vi "Process.vi"(8 "error in":errorcluster, 11 "MauiTemplate":refnum<class "SMO.UI.MAUI.BasicTemplate.lvclass">) -> (0 "error out":errorcluster, 3 "MauiTemplate out":refnum<class "SMO.UI.MAUI.BasicTemplate.lvclass">)   [LabVIEW 2019, in "SMO.UI.MAUI.BasicTemplate.lvclass"]
doc: "---------------------------------------------------------------\nJKI State Machine Objects™\nhttp://jki.net/state-machine-objects/\nCopyright (C) 2005-2015, JKI <info@jki.net>\nALL RIGHTS RESERVED"
uses:
  SMO.UI.MAUI.BasicTemplate.lvclass
  C:/Program Files (x86)/National Instruments/LabVIEW 2019/vi.lib/JKI/JKI SMO/SMO/SMO.lvclass
  C:/Users/patrick/Documents/GitHub/MAUI-Engine/lvsrc/Maui 1.0/SMO.UI.MAUI/SMO.UI.MAUI.lvclass
  C:/Program Files (x86)/National Instruments/LabVIEW 2019/vi.lib/JKI/JKI SMO/SMO.UI/SMO.UI.lvclass
  <vilib>/JKI/JKI SMO/SMO/Typedefs/Parent Call--Enum.ctl
  <vilib>/JKI/JKI SMO/SMO/SMO.lvclass/SMO.ctl
  Maui 1.0/SMO.UI.MAUI/Typedefs/PanelData.ctl
  <vilib>/JKI/JKI SMO/SMO/Private/ReftoDVR--SMO.vi
  Maui 1.0/SMO.UI.MAUI/SMO.UI.MAUI.lvclass
  <vilib>/JKI/JKI SMO/SMO/SMO.lvclass
  <vilib>/JKI/JKI SMO/SMO.UI/SMO.UI.lvclass
panel:
  out "Title":string
  in  "Right Ring":u16(ring)
  in  "Left Ring":u16(ring)
  # "For instructions on how to use the JKI State Machine Objects, examples and video tutorials, visit:\nhttp://jki.net/state-machine-objects/\n\nJKI State Machine Objects™\nhttp://jki.net/state-machine-objects/\nCopyright (C) 2005-2015, JKI <info@jki.net>\nALL RIGHTS RESERVED"
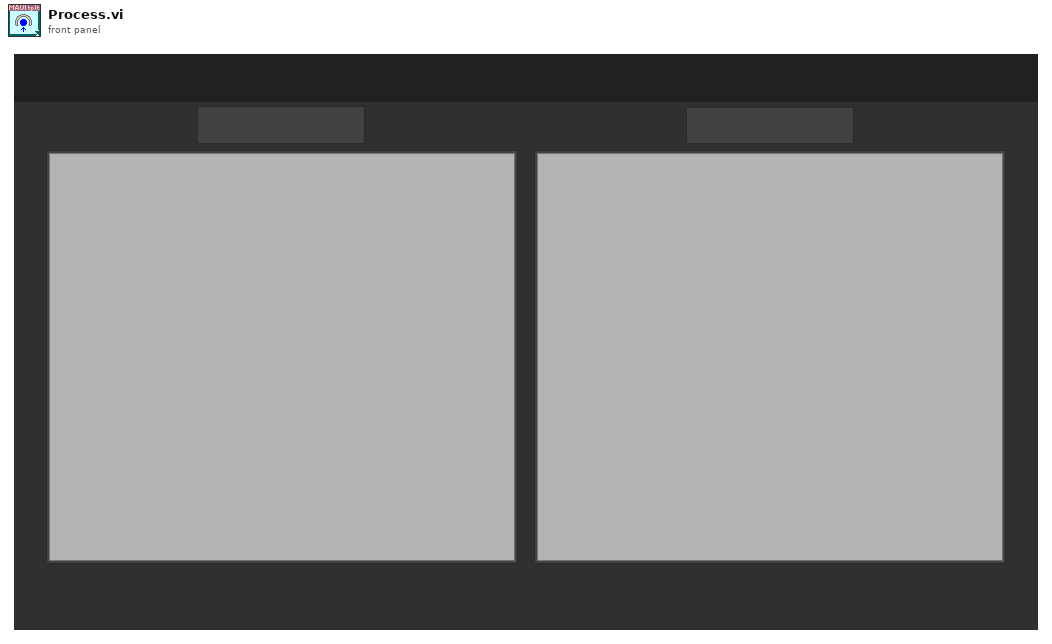
[diagram p1: front panel]
types:
  T1 = typedef "SMO.lvclass/Parent Call--Enum.ctl" = enum16{"Allows parent to run", "Does not request parent to run"}
  T2 = enum32{"invalid app kind", "Development System", "Run Time System", "Student Edition", "Embedded LabVIEW", "Evaluation", "Custom"}
  T3 = enum32{"Invalid", "Standard", "Closed", "Hidden", "Minimized", "Maximized"}
  T4 = enum32{"Bad", "Idle", "Run top level", "Running"}
  T5 = cluster{"Core":cluster{"Current VI Reference":refnum<vi>, "Close Panel on Exit?":bool, "error":errorcluster}, "MAUI":cluster{"Active Index":i32, "Panel Index":i32}, "Self Reference":refnum<class "SMO.UI.MAUI.BasicTemplate.lvclass">}
  T6 = cluster{"Current VI Reference":refnum<vi>, "Close Panel on Exit?":bool, "error":errorcluster}
  T7 = typedef "SMO.lvclass/Protected Events.ctl" = cluster{"StopProcesses":refnum<user-event>, "AbortProcesses":refnum<user-event>, "Config Changed":refnum<user-event>, "Dependency":refnum<user-event>}
  T8 = typedef "SMO.UI.MAUI.lvclass/PublicEvents--Cluster.ctl" = cluster{"ReadyForInfo ":refnum<user-event>}
  T9 = typedef "SMO.UI.MAUI.lvclass/PanelData.ctl" = cluster{"SubPanel":refnum<vi>, "Ring":refnum<vi>, "Active":i32}
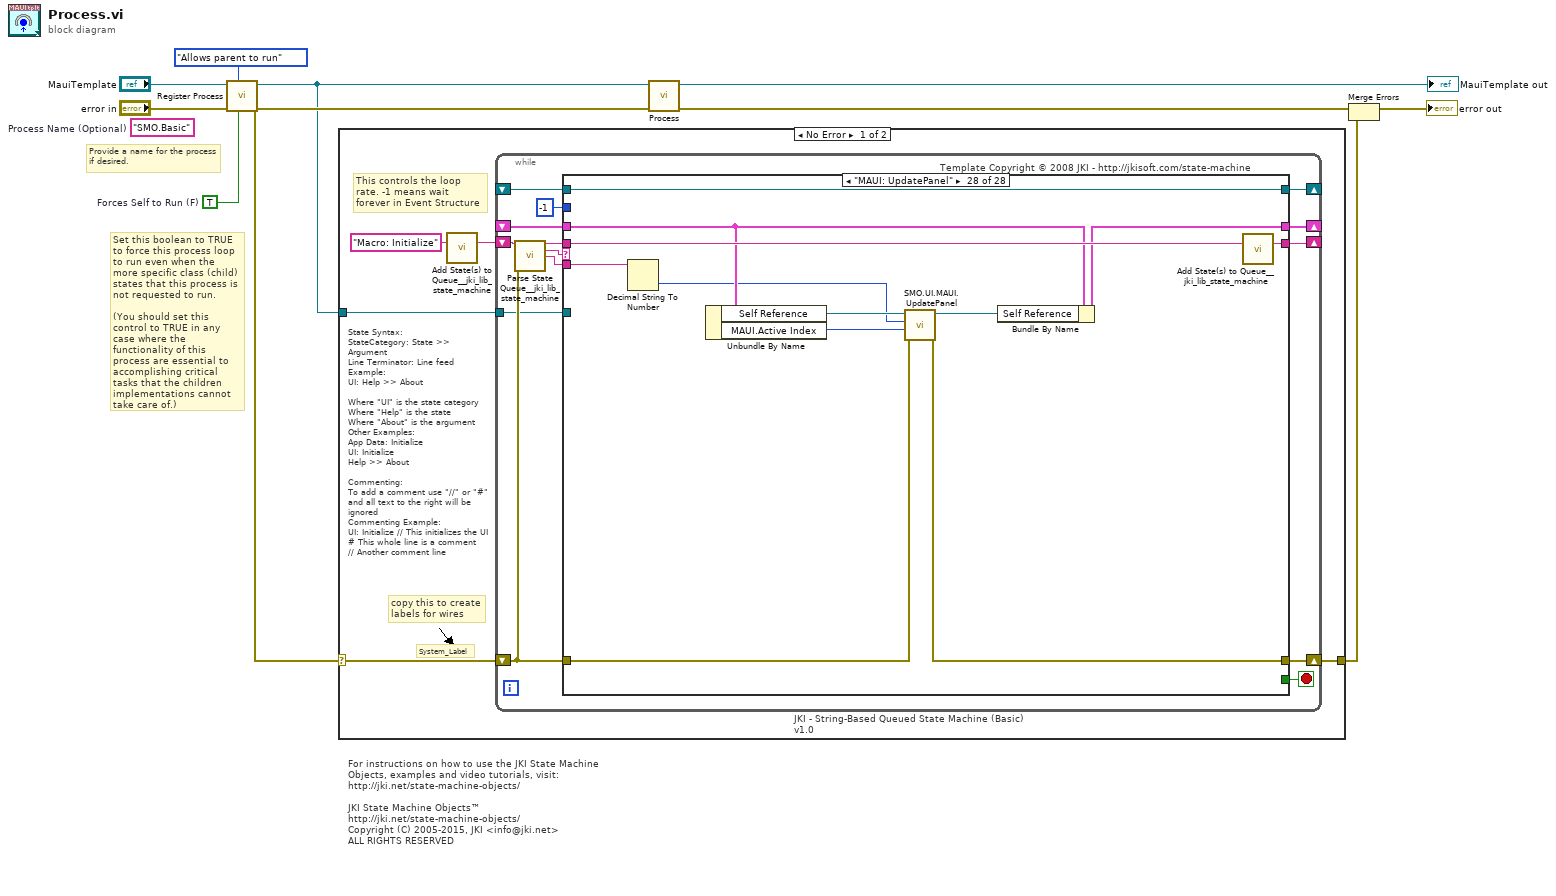
[diagram p0: block diagram]
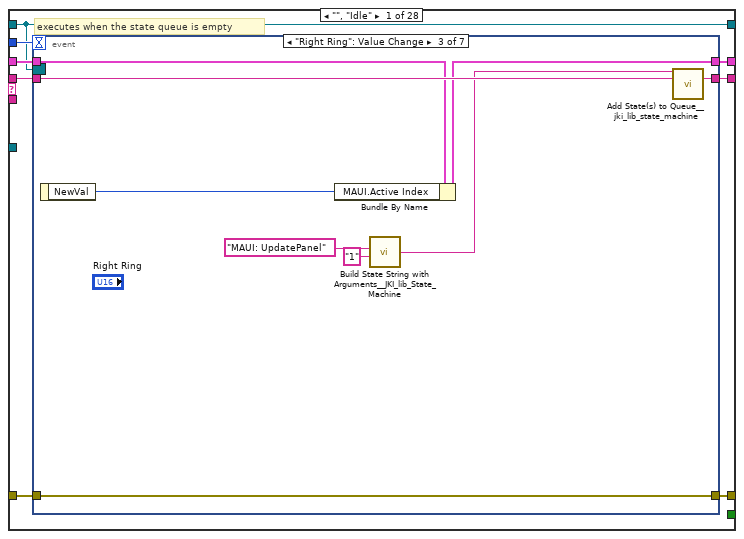
[diagram p2: hidden frame]
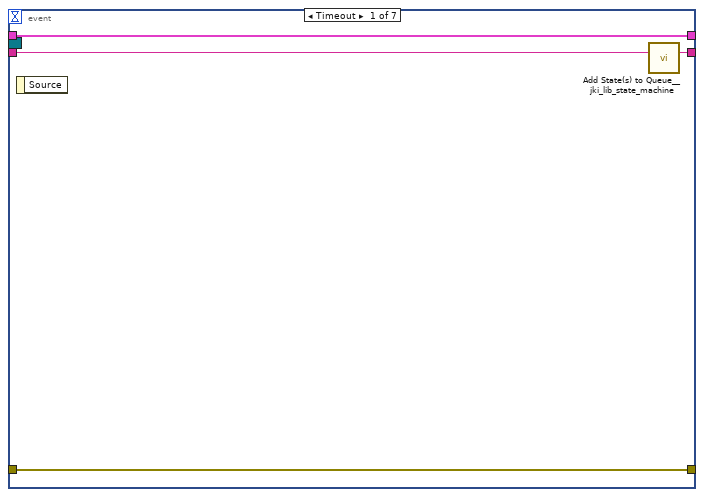
[diagram p3: hidden frame]
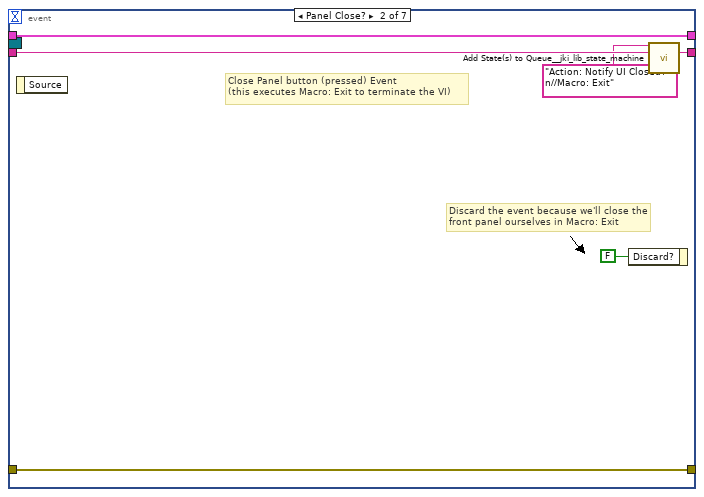
[diagram p4: hidden frame]
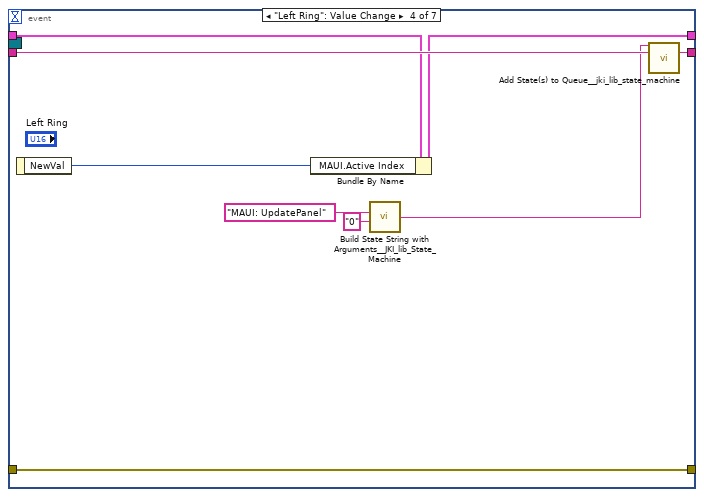
[diagram p5: hidden frame]
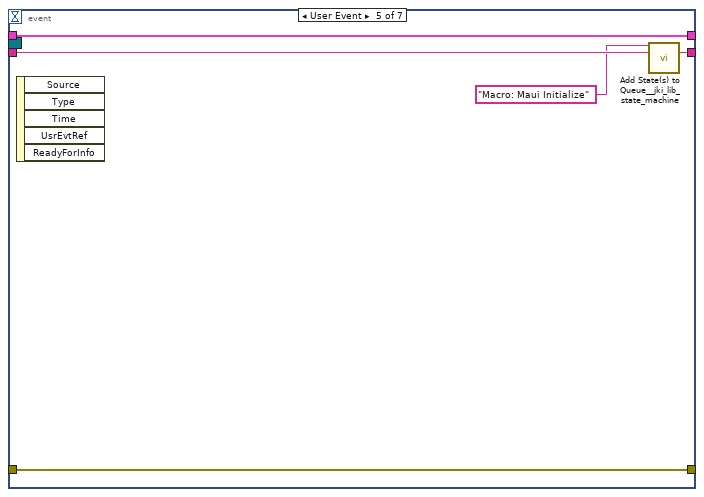
[diagram p6: hidden frame]
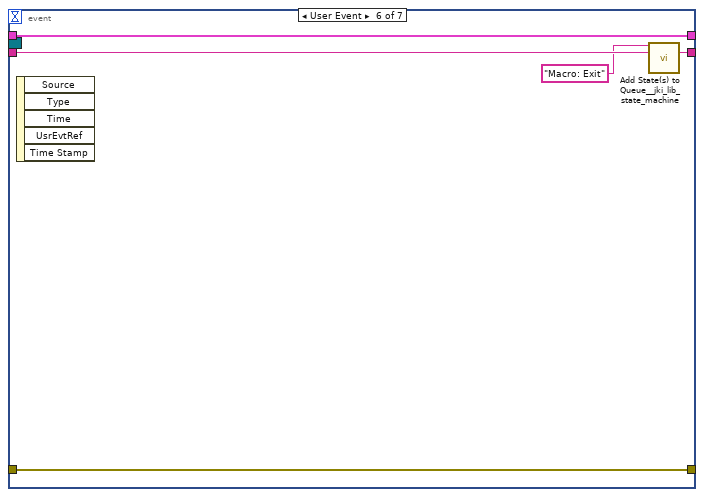
[diagram p7: hidden frame]
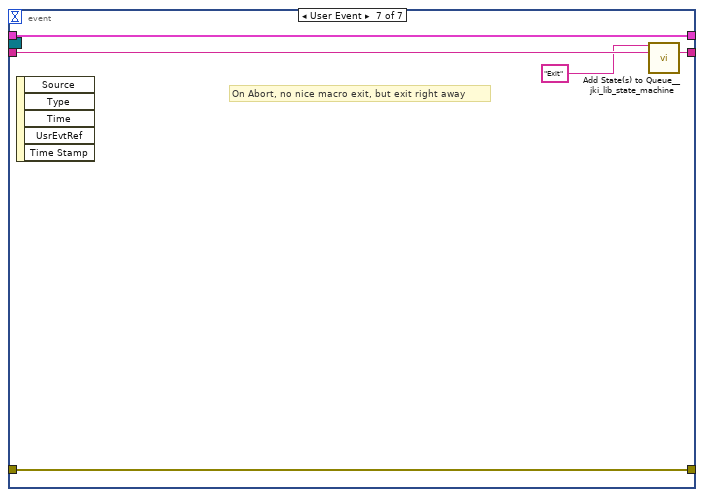
[diagram p8: hidden frame]
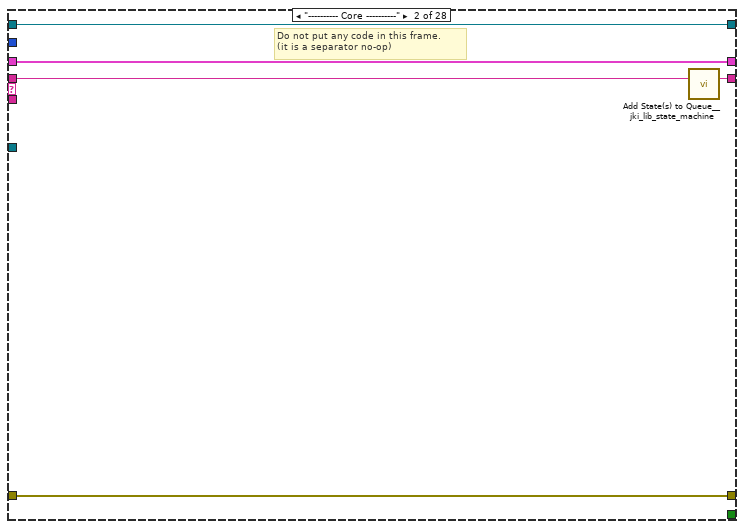
[diagram p9: hidden frame]
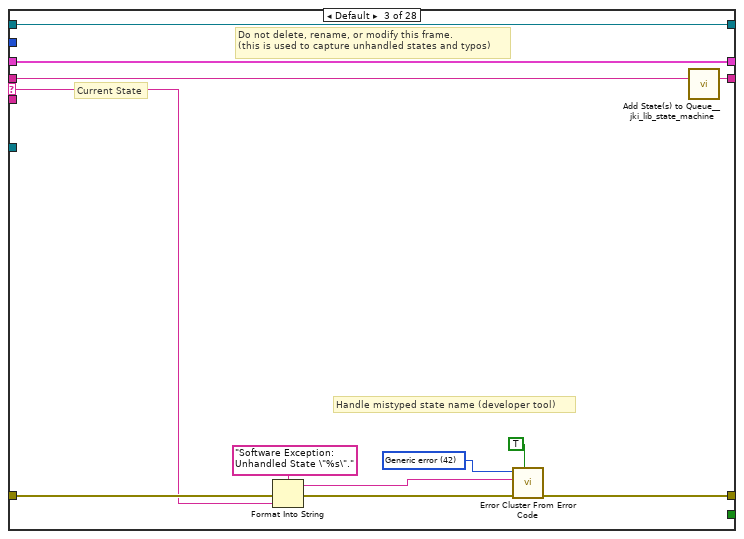
[diagram p10: hidden frame]
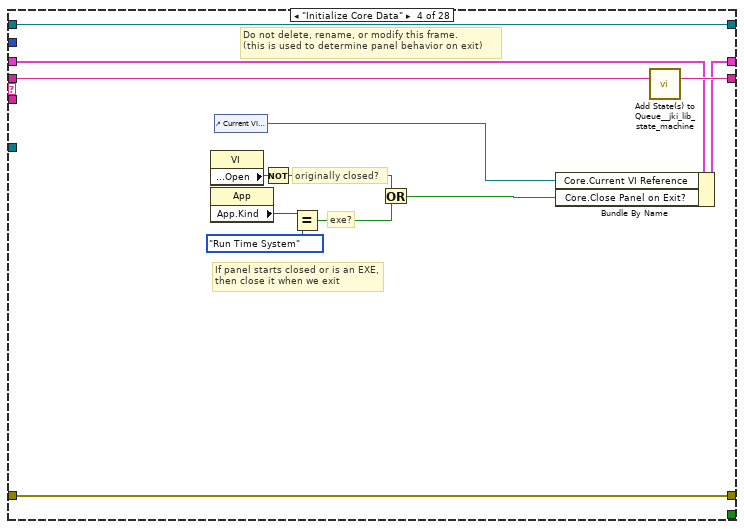
[diagram p11: hidden frame]
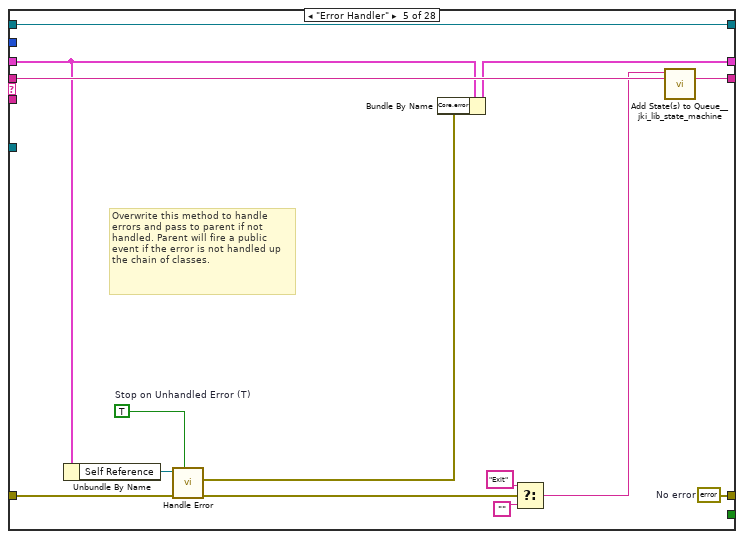
[diagram p12: hidden frame]
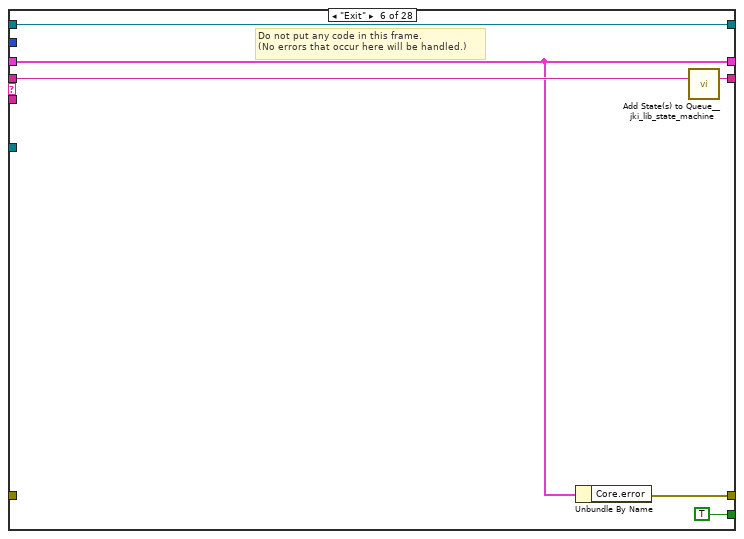
[diagram p13: hidden frame]
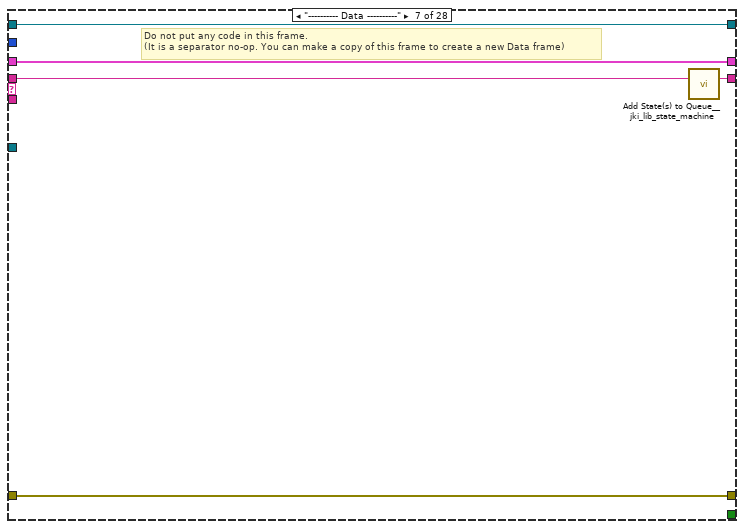
[diagram p14: hidden frame]
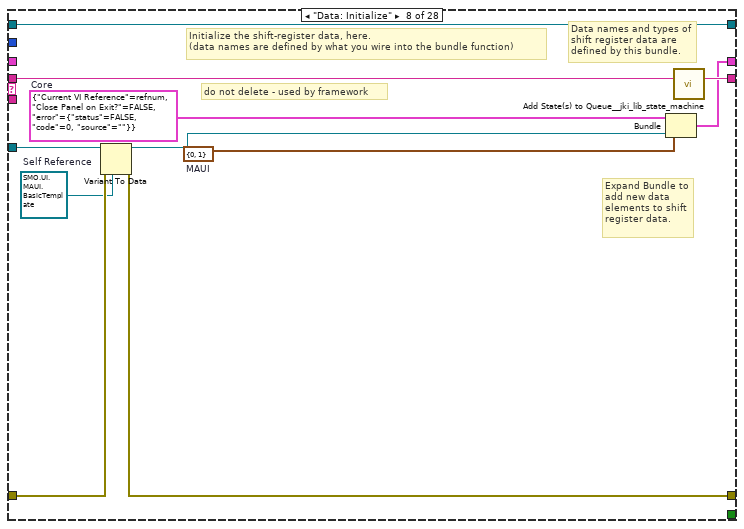
[diagram p15: hidden frame]
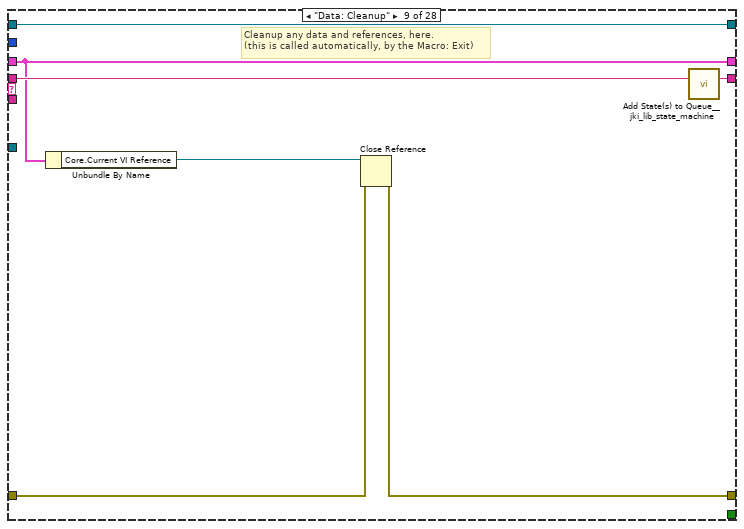
[diagram p16: hidden frame]
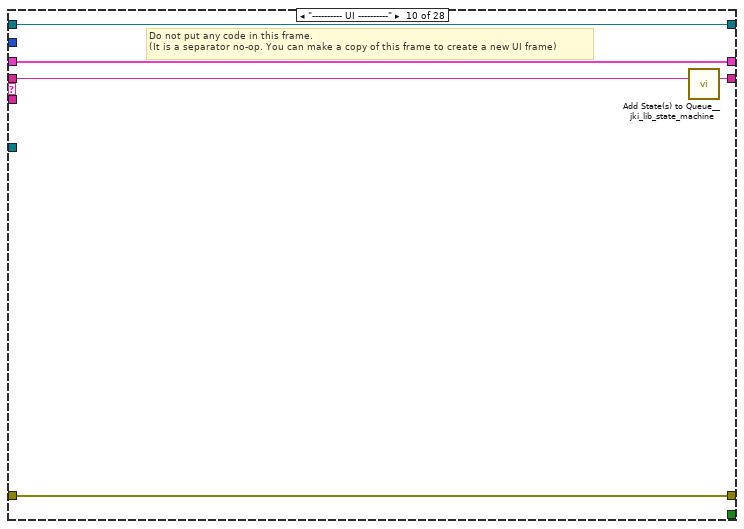
[diagram p17: hidden frame]
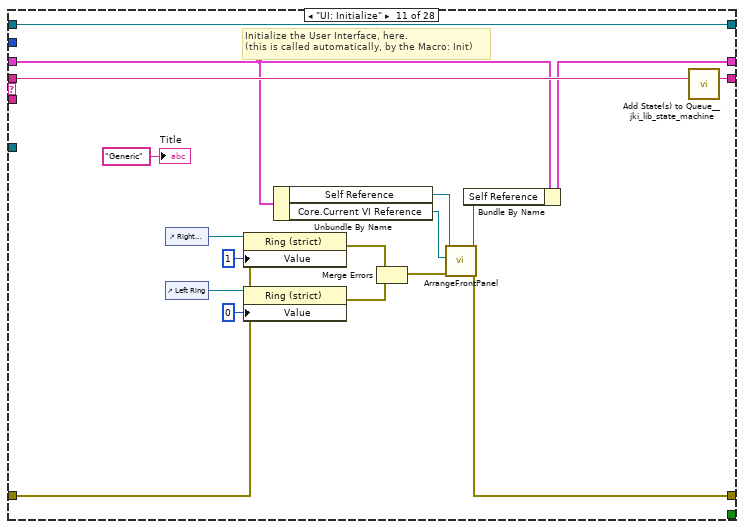
[diagram p18: hidden frame]
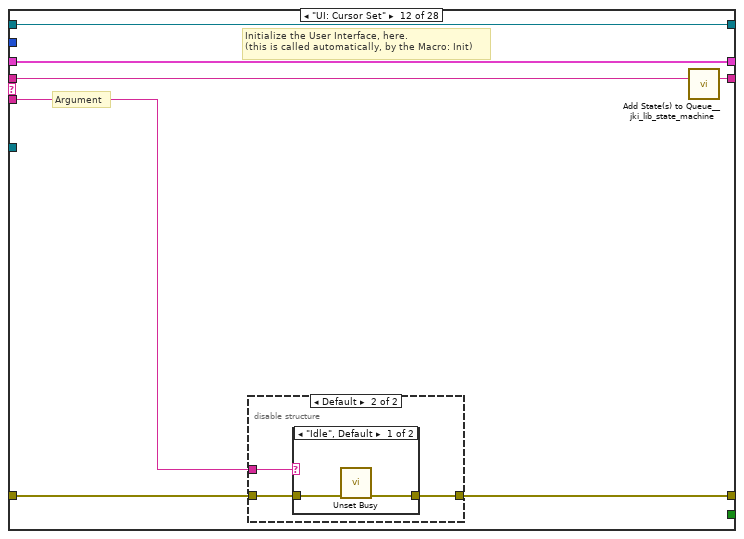
[diagram p19: hidden frame]
diagram:
  w2 = TRUE  # Forces Self to Run (F)
  (unwired) "SMO.Basic"  # Process Name (Optional)
  # "Provide a name for the process\nif desired."
  # "Set this boolean to TRUE to force this process loop to run even when the more specific class (child) states that this process is not requested to run.\n\n(You should set this control to TRUE in any case where the functionality of this process are essential to accomplishing critical tasks that the children implementations cannot take care of.)"
  # "For instructions on how to use the JKI State Machine Objects, examples and video tutorials, visit:\nhttp://jki.net/state-machine-objects/\n\nJKI State Machine Objects™\nhttp://jki.net/state-machine-objects/\nCopyright (C) 2005-2015, JKI <info@jki.net>\nALL RIGHTS RESERVED"
  n1 = call <vilib>:"Register Process.vi"("Forces Self to Run (F)"=w2, "Parent Call"=Parent_Call--Enum."Allows parent to run", "error in (no error)"="error in", "SMO"="MauiTemplate") -> ("error out"=w7:errorcluster, "SMO out"=w1:refnum<class "SMO.UI.MAUI.BasicTemplate.lvclass">)  [unwired: 6 in]
  n2 = case shown="No Error" w7 {
    selector: w7 -> [w12 w360]
    tunnel: w1 -> [w13 _]
    tunnel: [w11 w360] -> w4
    frame No Error {
      # "State Syntax:\nStateCategory: State >> Argument\nLine Terminator: Line feed\nExample:\nUI: Help >> About\n\nWhere \"UI\" is the state category\nWhere \"Help\" is the state\nWhere \"About\" is the argument\nOther Examples:\nApp Data: Initialize\nUI: Initialize\nHelp >> About\n\nCommenting:\nTo add a comment use \"//\" or \"#\" and all text to the right will be ignored\nCommenting Example:\nUI: Initialize // This initializes the UI\n# This whole line is a comment\n// Another comment line"
      # "copy this to create labels for wires"
      # "This controls the loop rate. -1 means wait forever in Event Structure"
      # "System_Label"
      n3 = call <vilib>:"Add State(s) to Queue__jki_lib_state_machine.vi"("State(s) in (\"\")"="Macro: Initialize") -> ("States Out"=w15:string)  [unwired: 14 in]
      n4 = while "JKI - String-Based Queued State Machine (Basic) v1.0" {
        shift-right: [w22] -> _
        shift-left: _ -> [w21]
        shift-right: [w25] -> w11
        shift-left: w12 -> [w19]
        shift-right: [w24] -> _
        shift-left: w15 -> [w26]
        tunnel: w13 -> [w18]
        shift-right: [w17] -> _
        shift-left: _ -> [w16]
        stop <- w23 stop-if-true
        # "Template Copyright © 2008 JKI - http://jkisoft.com/state-machine"
        n5 = call <vilib>:"Parse State Queue__jki_lib_state_machine.vi"("State Queue"=w26, "Error In (no error)"=w19) -> ("Remaining States"=w28:string, "Current State"=w29:string, "Arguments"=w27:string)  [unwired: 11 in]
        n6 = case shown="\"MAUI: UpdatePanel\"" w29 {
          selector: w29 -> [_ _ w87 _ _ _ _ _ _ _ _ _ _ _ _ _ _ _ _ _ _ _ _ _ _ _ _ _]
          tunnel: w28 -> [w37 w85 w91 w110 w124 w130 w135 w146 w153 w158 w176 w183 w199 w231 w245 w251 w265 w270 w281 w286 w298 w304 w309 w316 w323 w328 w347 w359]
          tunnel: w27 -> [_ _ _ _ _ _ _ _ _ _ _ w177 w193 _ _ _ _ _ _ _ _ _ _ _ _ _ _ w354]
          tunnel: w21 -> [w35 w82 w89 w101 w118 w126 w132 _ w148 w155 w171 w181 w195 w228 w241 w248 w256 w267 w278 w283 w296 w302 w307 w313 w319 w326 w344 w356]
          tunnel: [w34 w83 w93 w107 w119 w125 w133 w142 w149 w156 w160 w178 w196 w229 w243 w249 w263 w268 w272 w284 w292 w300 w305 w310 w320 w324 w329 w352] -> w25
          tunnel: w19 -> [w33 w83 w92 w107 w120 _ w133 w143 w150 w156 w166 w179 w197 w229 w243 w249 w263 w268 w273 w284 w293 w300 w305 w311 w320 w324 w333 w353]
          tunnel: [w36 w84 w90 w109 w123 w129 w134 w145 w152 w157 w175 w182 w198 w230 w244 w250 w264 w269 w280 w285 w297 w303 w308 w315 w322 w327 w346 w358] -> w24
          tunnel: [_ _ _ _ _ TRUE _ _ _ _ _ _ _ _ _ _ _ _ _ _ _ _ _ _ _ _ _ _] -> w23
          tunnel: [w32 w82 w89 w108 w117 w126 w132 w144 w148 w155 w170 w181 w195 w228 w241 w248 w256 w267 w278 w283 w296 w302 w307 w313 w318 w326 w343 w355] -> w22
          tunnel: -1 ("Timeout") -> [w31 _ _ _ _ _ _ _ _ _ _ _ _ _ _ _ _ _ _ _ _ _ _ _ _ _ _ _]
          tunnel: w18 -> [_ _ _ _ _ _ _ w140 _ _ _ _ _ _ _ _ _ _ _ _ _ _ _ _ _ _ _ _]
          tunnel: [w30 w81 w86 w98 w122 w127 w131 w139 w147 w154 w174 w180 w192 w227 w242 w247 w257 w266 w279 w282 w295 w301 w306 w314 w321 w325 w345 w357] -> w17
          tunnel: w16 -> [w30 w81 w86 w98 w122 w127 w131 w139 w147 w154 w174 w180 w192 w227 w242 w247 w257 w266 w279 w282 _ w301 w306 w314 w321 w325 w345 w357]
          frame "", "Idle" {
            # "executes when the state queue is empty"
            n7 = event shown="[2] \"Right Ring\": Value Change" {
              selector: w30 -> [_ _ _ _ _ _ _]
              dyn-events: _ -> [_ _ _ _ _ _ _]
              timeout: w31 -> [_ _ _ _ _ _ _]
              tunnel: w37 -> [w41 w47 w56 w65 w70 w75 w80]
              tunnel: [w40 w46 w55 w64 w69 w74 w79] -> w36
              tunnel: w35 -> [w39 w44 w53 w62 w68 w72 w77]
              tunnel: [w38 w45 w54 w63 w67 w73 w78] -> w34
              tunnel: w33 -> [w38 w45 w54 w63 w67 w73 w78]
              tunnel: [w39 w44 w52 w61 w68 w72 w77] -> w32
              event Timeout {
                n8 = event-data() -> ()  [unwired: 1 in, 1 out]
                n9 = call <vilib>:"Add State(s) to Queue__jki_lib_state_machine.vi"("State(s) in (\"\")"=w41) -> ("States Out"=w40:string)  [unwired: 14 in]
              }
              event Panel Close? {
                # "Discard the event because we'll close the front panel ourselves in Macro: Exit"
                # "Close Panel button (pressed) Event\n(this executes Macro: Exit to terminate the VI)"
                n10 = event-data() -> ()  [unwired: 1 in, 1 out]
                n11 = event-data("Discard?"=FALSE) -> ()  [unwired: 1 in, 1 out]
                n12 = call <vilib>:"Add State(s) to Queue__jki_lib_state_machine.vi"("State(s) in Front (\"\")"="Action: Notify UI Closed\n//Macro: Exit", "State(s) in (\"\")"=w47) -> ("States Out"=w46:string)  [unwired: 13 in]
              }
              event "Right Ring": Value Change {
                n13 = event-data() -> ("NewVal"=w51:u16)  [unwired: 1 in]
                n14 = Bundle By Name(cluster=w53, "MAUI.Active Index"=w51) -> (w52:T5)
                n15 = call <vilib>:"Build State String with Arguments__JKI_lib_State_Machine.vi"("Arguments (\"\")"="1" ("Arguments (\"\")"), "State"="MAUI: UpdatePanel") -> ("State with Arguments"=w48:string)  [unwired: 4 in]
                n16 = call <vilib>:"Add State(s) to Queue__jki_lib_state_machine.vi"("State(s) in Front (\"\")"=w48, "State(s) in (\"\")"=w56) -> ("States Out"=w55:string)  [unwired: 13 in]
              }
              event "Left Ring": Value Change {
                n17 = event-data() -> ("NewVal"=w60:u16)  [unwired: 1 in]
                n18 = Bundle By Name(cluster=w62, "MAUI.Active Index"=w60) -> (w61:T5)
                n19 = call <vilib>:"Build State String with Arguments__JKI_lib_State_Machine.vi"("Arguments (\"\")"="0" ("Arguments (\"\")"), "State"="MAUI: UpdatePanel") -> ("State with Arguments"=w57:string)  [unwired: 4 in]
                n20 = call <vilib>:"Add State(s) to Queue__jki_lib_state_machine.vi"("State(s) in Front (\"\")"=w57, "State(s) in (\"\")"=w65) -> ("States Out"=w64:string)  [unwired: 13 in]
              }
              event User Event {
                n21 = event-data() -> ()  [unwired: 1 in, 5 out]
                n22 = call <vilib>:"Add State(s) to Queue__jki_lib_state_machine.vi"("State(s) in Front (\"\")"="Macro: Maui Initialize", "State(s) in (\"\")"=w70) -> ("States Out"=w69:string)  [unwired: 13 in]
              }
              event User Event {
                n23 = event-data() -> ()  [unwired: 1 in, 5 out]
                n24 = call <vilib>:"Add State(s) to Queue__jki_lib_state_machine.vi"("State(s) in Front (\"\")"="Macro: Exit", "State(s) in (\"\")"=w75) -> ("States Out"=w74:string)  [unwired: 13 in]
              }
              event User Event {
                # "On Abort, no nice macro exit, but exit right away"
                n25 = event-data() -> ()  [unwired: 1 in, 5 out]
                n26 = call <vilib>:"Add State(s) to Queue__jki_lib_state_machine.vi"("State(s) in Front (\"\")"="Exit", "State(s) in (\"\")"=w80) -> ("States Out"=w79:string)  [unwired: 13 in]
              }
            }
          }
          frame "---------- Core ----------" {
            # "Do not put any code in this frame.\n(it is a separator no-op)"
            n27 = call <vilib>:"Add State(s) to Queue__jki_lib_state_machine.vi"("State(s) in (\"\")"=w85) -> ("States Out"=w84:string)  [unwired: 14 in]
          }
          frame Default {
            w96 = 42 items=["No error", "Argument error", "Memory is full", "Out of zone", "End of file", "File already open", "Generic file I/O error", "File not found", "File permission error", "Disk is full", "Duplicate path", "Too many files open", "System feature not enabled", "Resource file not found", "Cannot add resource", "Resource not found", "Image not found", "Image memory error", "Pen does not exist", "Config type invalid", "Config token not found", "Config parse error", "Config memory error", "Bad external code format", "Bad external code offset", "External code not present", "Null window", "Destroy window error", "Null menu", "Print aborted", "Bad print record", "Print driver error", "Windows error during printing", "Memory error during printing", "Print dialog error", "Generic print error", "Invalid device refnum", "Device not found", "Device parameter error", "Device unit error", "Cannot open device", "Device call aborted", "Generic error", "Cancelled by user", "Object ID too low", "Object ID too high", "Object not in heap", "Unknown heap", "Unknown object (invalid DefProc)", "Unknown object (DefProc not in table)", "Message out of range", "Invalid (null) method", "Unknown message", "Manager call not supported", "Bad address", "Network operation in progress", "Network operation timed out", "Connection is busy", "Network attribute not supported", "Network error", "Address in use", "System out of memory", "Connection aborted", "Connection refused", "Not connected", "Already connected", "Connection closed", "Initialization error (interapplication manager)", "Bad occurrence", "Wait on unbound occurrence handler", "Occurrence queue overflow", "Datalog type conflict", "Unused", "Unrecognized type (interapplication manager)", "Memory corrupt", "Failed to make temporary DLL", "Old CIN version", "Drag socket not found", "Failed to load drop-object", "Failed to register OLE object", "Failed to release OLE object", "Format specifier type mismatch", "Unknown format specifier", "Too few format specifiers", "Too many format specifiers", "Scan failed", "Newer CIN version", "Error converting to variant", "Runtime menu error", "Password tampered", "Variant attribute not found", "Incompatible variant data type", "Event data is not available", "Event Store is not present", "Occurrence is not found", "Event Queue is not created", "Event info is not available", "Refnum passed is NULL", "Error retrieving Class GUID", "Error retrieving CoClass GUID", "Error retrieving TypeLib GUID.", "Bad built application magic bytes.", "Specific driver is different from the specific driver associated with the Logical Name.", "There is no session opened to the class driver.", "Max Error", "MAX - Error with config objects", "MAX - Error loading configuration", "MAX - Group not supported"]
            # "Current State"
            # "Do not delete, rename, or modify this frame.\n(this is used to capture unhandled states and typos)"
            # "Handle mistyped state name (developer tool)"
            n28 = Format Into String(format string="Software Exception: Unhandled State \"%s\"." ("message"), error in=w92, w87) -> (resulting string=w95:string, error out=w94:errorcluster)  [unwired: 1 in]
            n29 = call <vilib>:"Error Cluster From Error Code.vi"("show call chain? (False)"=TRUE, "error in (no error)"=w94, "error message (\"\")"=w95, "error code (0)"=w96) -> ("error out"=w93:errorcluster)  [unwired: 5 in]
            n30 = call <vilib>:"Add State(s) to Queue__jki_lib_state_machine.vi"("State(s) in (\"\")"=w91) -> ("States Out"=w90:string)  [unwired: 14 in]
          }
          frame "Initialize Core Data" {
            # "Do not delete, rename, or modify this frame.\n(this is used to determine panel behavior on exit)"
            # "originally closed?"
            # "exe?"
            # "If panel starts closed or is an EXE, then close it when we exit"
            n31 = property class="VI"() -> ("Front Panel.Open"=w106:bool)  [unwired: 2 in, 2 out]
            n32 = property class="App"() -> ("App.Kind"=w105:T2)  [unwired: 2 in, 2 out]
            n33 = control-ref of="Current VI Reference"() -> (w99:refnum<vi>)
            n34 = Not(x=w106) -> (.not. x?=w103:bool)
            n35 = Equal?(x=w105, y=T2."Run Time System" ("Application:Kind")) -> (x = y?=w102:bool)
            n36 = Or(x=w103, y=w102) -> (x .or. y?=w100:bool)
            n37 = Bundle By Name(cluster=w101, "Core.Current VI Reference"=w99, "Core.Close Panel on Exit?"=w100) -> (w108:T5)
            n38 = call <vilib>:"Add State(s) to Queue__jki_lib_state_machine.vi"("State(s) in (\"\")"=w110) -> ("States Out"=w109:string)  [unwired: 14 in]
          }
          frame "Error Handler" {
            w111 = TRUE  # Stop on Unhandled Error (T)
            w119 = errorcluster {"status"=FALSE, "code"=0, "source"=""}  # No error
            # "Overwrite this method to handle errors and pass to parent if not handled. Parent will fire a public event if the error is not handled up the chain of classes."
            n39 = Unbundle By Name(w118) -> ("Self Reference"=w121:refnum<class "SMO.UI.MAUI.BasicTemplate.lvclass">)
            n40 = call-dynamic "Handle Error.vi"("Stop on Unhandled Error (T)"=w111, "error in"=w120, "SMO"=w121) -> ("handling error"=w112:errorcluster, "Unhandled error"=w115:errorcluster)  [unwired: 6 in, 1 out]
            n41 = Bundle By Name(cluster=w118, "Core.error"=w115) -> (w117:T5)
            n42 = Select(t="Exit", s=w112, f="") -> (s? t:f=w116:string)
            n43 = call <vilib>:"Add State(s) to Queue__jki_lib_state_machine.vi"("State(s) in Front (\"\")"=w116, "State(s) in (\"\")"=w124) -> ("States Out"=w123:string)  [unwired: 13 in]
          }
          frame "Exit" {
            # "Do not put any code in this frame.\n(No errors that occur here will be handled.)"
            n44 = Unbundle By Name(w126) -> ("Core.error"=w125:errorcluster)
            n45 = call <vilib>:"Add State(s) to Queue__jki_lib_state_machine.vi"("State(s) in (\"\")"=w130) -> ("States Out"=w129:string)  [unwired: 14 in]
          }
          frame "---------- Data ----------" {
            # "Do not put any code in this frame.\n(It is a separator no-op. You can make a copy of this frame to create a new Data frame)"
            n46 = call <vilib>:"Add State(s) to Queue__jki_lib_state_machine.vi"("State(s) in (\"\")"=w135) -> ("States Out"=w134:string)  [unwired: 14 in]
          }
          frame "Data: Initialize" {
            w137 = cluster{"Active Index":i32, "Panel Index":i32} {"Active Index"=0, "Panel Index"=1}  # MAUI
            w138 = T6 {"Current VI Reference"=refnum, "Close Panel on Exit?"=FALSE, "error"={"status"=FALSE, "code"=0, "source"=""}}  # Core
            w141 = refnum<class "SMO.UI.MAUI.BasicTemplate.lvclass"> refnum  # Self Reference
            # "do not delete - used by framework"
            # "Expand Bundle to add new data elements to shift register data."
            # "Data names and types of shift register data are defined by this bundle."
            # "Initialize the shift-register data, here.\n(data names are defined by what you wire into the bundle function)"
            n47 = Variant To Data(error in=w143, type=w141, Variant=w140) -> (data=w136:refnum<class "SMO.UI.MAUI.BasicTemplate.lvclass">, error out=w142:errorcluster)
            n48 = Bundle("Core"=w138, "MAUI"=w137, "Self Reference"=w136) -> (w144:T5)  [unwired: 1 in]
            n49 = call <vilib>:"Add State(s) to Queue__jki_lib_state_machine.vi"("State(s) in (\"\")"=w146) -> ("States Out"=w145:string)  [unwired: 14 in]
          }
          frame "Data: Cleanup" {
            # "Cleanup any data and references, here.\n(this is called automatically, by the Macro: Exit)"
            n50 = Unbundle By Name(w148) -> ("Core.Current VI Reference"=w151:refnum<vi>)
            n51 = Close Reference(reference=w151, error in (no error)=w150) -> (error out=w149:errorcluster)
            n52 = call <vilib>:"Add State(s) to Queue__jki_lib_state_machine.vi"("State(s) in (\"\")"=w153) -> ("States Out"=w152:string)  [unwired: 14 in]
          }
          frame "---------- UI ----------" {
            # "Do not put any code in this frame.\n(It is a separator no-op. You can make a copy of this frame to create a new UI frame)"
            n53 = call <vilib>:"Add State(s) to Queue__jki_lib_state_machine.vi"("State(s) in (\"\")"=w158) -> ("States Out"=w157:string)  [unwired: 14 in]
          }
          frame "UI: Initialize" {
            # "Initialize the User Interface, here.\n(this is called automatically, by the Macro: Init)"
            n54 = control-ref of="Right Ring"() -> (w173:refnum<vi>)
            n55 = control-ref of="Left Ring"() -> (w168:refnum<vi>)
            n56 = property class="Ring (strict)"(reference=w173, error in=w166, "Value"=u16 1) -> (error out=w164:errorcluster)  [unwired: 1 out]
            n57 = property class="Ring (strict)"(reference=w168, error in=w166, "Value"=u16 0) -> (error out=w165:errorcluster)  [unwired: 1 out]
            n58 = Unbundle By Name(w171) -> ("Self Reference"=w163:refnum<class "SMO.UI.MAUI.BasicTemplate.lvclass">, "Core.Current VI Reference"=w162:refnum<vi>)
            n59 = Merge Errors(w164, w165) -> (w161:errorcluster)
            n60 = call "ArrangeFrontPanel.vi"("error in (no error)"=w161, "This VI"=w162, "MAUI in"=w163) -> ("error out"=w160:errorcluster, "MAUI out"=w159:refnum<class "SMO.UI.MAUI.BasicTemplate.lvclass">)  [unwired: 7 in]
            n61 = Bundle By Name(cluster=w171, "Self Reference"=w159) -> (w170:T5)
            n62 = call <vilib>:"Add State(s) to Queue__jki_lib_state_machine.vi"("State(s) in (\"\")"=w176) -> ("States Out"=w175:string)  [unwired: 14 in]
            "Title" <- "Generic" ("Title")
          }
          frame "UI: Cursor Set" {
            # "Argument"
            # "Initialize the User Interface, here.\n(this is called automatically, by the Macro: Init)"
            n63 = disable-structure shown="Default" {
              disable-tunnel: w179 -> [w184 w187]
              disable-tunnel: [w184 w186] -> w178
              disable-tunnel: w177 -> [_ w185]
              frame condition #0 {
              }
              frame condition #1 (active) {
                n64 = case shown="\"Idle\", Default" w185 {
                  tunnel: w187 -> [w189 w191]
                  tunnel: [w188 w190] -> w186
                  frame "Idle", Default {
                    n65 = call <vilib>:"Unset Busy.vi"("error in (no error)"=w189) -> ("error out"=w188:errorcluster)  [unwired: 10 in]
                  }
                  frame "Busy" {
                    n66 = call <vilib>:"Set Busy.vi"("error in (no error)"=w191) -> ("error out"=w190:errorcluster)  [unwired: 9 in, 1 out]
                  }
                }
              }
            }
            n67 = call <vilib>:"Add State(s) to Queue__jki_lib_state_machine.vi"("State(s) in (\"\")"=w183) -> ("States Out"=w182:string)  [unwired: 14 in]
          }
          frame "UI: Front Panel State" {
            # "Argument"
            # "Set Front Panel Open or Closed\n(Usage: \"UI: Front Panel State >> Open|Close\")"
            n68 = Unbundle By Name(w195) -> ("Core.Current VI Reference"=w194:refnum<vi>)
            n69 = disable-structure shown="Default" {
              disable-tunnel: w197 -> [w203 w226]
              disable-tunnel: [w202 w226] -> w196
              disable-tunnel: w194 -> [w201 _]
              disable-tunnel: w193 -> [w200 _]
              frame condition #0 (active) {
                n70 = case shown="\"Close\"" w200 {
                  tunnel: w203 -> [w207 w220]
                  tunnel: [w209 w221] -> w202
                  tunnel: w201 -> [w208 w218]
                  frame "Open", Default {
                    n71 = property class="VI"(reference=w208, error in=w207) -> (reference out=w205:refnum<vi>, error out=w206:errorcluster, "FP.State"=w204:T3)
                    n72 = case shown="\"Closed\"" w204 {
                      tunnel: [w212 w215] -> w209
                      tunnel: w206 -> [w211 w215]
                      tunnel: w205 -> [w210 _]
                      frame "Closed" {
                        n73 = invoke class="VI" method="FP.Open"(reference=w210, error in=w211, "Activate"=TRUE, "State"=T3."Standard") -> (error out=w212:errorcluster)  [unwired: 1 in, 4 out]
                      }
                      frame Default {
                      }
                    }
                  }
                  frame "Close" {
                    n74 = property class="VI"(reference=w218, error in=w220) -> (reference out=w217:refnum<vi>, error out=w219:errorcluster, "FP.State"=w216:T3)
                    n75 = case shown="Default" w216 {
                      tunnel: [w222 w225] -> w221
                      tunnel: w219 -> [w222 w224]
                      tunnel: w217 -> [_ w223]
                      frame "Invalid", "Closed" {
                      }
                      frame Default {
                        n76 = invoke class="VI" method="FP.Close"(reference=w223, error in=w224) -> (error out=w225:errorcluster)  [unwired: 1 in, 2 out]
                      }
                    }
                  }
                }
              }
              frame condition #1 {
              }
            }
            n77 = call <vilib>:"Add State(s) to Queue__jki_lib_state_machine.vi"("State(s) in (\"\")"=w199) -> ("States Out"=w198:string)  [unwired: 14 in]
          }
          frame "---------- Macro ----------" {
            # "Do not put any code in this frame.\n(It is a separator no-op. You can make a copy of this frame to create a new Macro frame)"
            n78 = call <vilib>:"Add State(s) to Queue__jki_lib_state_machine.vi"("State(s) in (\"\")"=w231) -> ("States Out"=w230:string)  [unwired: 14 in]
          }
          frame "Macro: Initialize" {
            w236 = "UI: Initialize\nUI: Front Panel State >> Open"  # UI: Initialize UI: Front Panel State >> Open
            w232 = "Process: Sync"
            # "Initialization Macro\n(This is called once, when the VI starts)"
            n79 = control-ref of="This VI"() -> (w234:refnum<vi>)
            n80 = property class="VI"(reference=w234) -> ("Exec.State"=w233:T4)  [unwired: 1 in, 2 out]
            n81 = Equal?(x=w233, y=T4."Run top level") -> (x = y?=w239:bool)
            n82 = Select(t=w232, s=w239, f="") -> ()  [unwired: 1 out]
            n83 = call <vilib>:"Add State(s) to Queue__jki_lib_state_machine.vi"("State(s) in Front (\"\")"="Data: Initialize\nInitialize Core Data\nEvents: Register", "State(s) in (\"\")"=w232, "State(s) at Back (\"\")"=w236) -> ("States Out"=w235:string)  [unwired: 12 in]
            n84 = call <vilib>:"Add State(s) to Queue__jki_lib_state_machine.vi"("State(s) in Front (\"\")"=w235, "State(s) in (\"\")"=w245) -> ("States Out"=w244:string)  [unwired: 13 in]
          }
          frame "Macro: Maui Initialize" {
            # "Do not put any code in this frame.\n(It is a separator no-op. You can make a copy of this frame to create a new Macro frame)"
            n85 = call <vilib>:"Add State(s) to Queue__jki_lib_state_machine.vi"("State(s) in Front (\"\")"="MAUI: SendPanelData", "State(s) in (\"\")"=w251) -> ("States Out"=w250:string)  [unwired: 13 in]
          }
          frame "Macro: Exit" {
            # "Exit Macro\n(This is called once, when the VI exits)"
            n86 = Unbundle By Name(w256) -> ("Core.Close Panel on Exit?"=w262:bool)
            n87 = Select(t="UI: Front Panel State >> Close", s=w262, f="") -> (s? t:f=w259:string)
            n88 = call <vilib>:"Add State(s) to Queue__jki_lib_state_machine.vi"("State(s) in Front (\"\")"="Data: Cleanup\nEvents: Unregister", "State(s) in (\"\")"="Process: Sync", "State(s) at Back (\"\")"="Exit") -> ("States Out"=w253:string)  [unwired: 12 in]
            n89 = call <vilib>:"Add State(s) to Queue__jki_lib_state_machine.vi"("State(s) in (\"\")"=w259, "State(s) at Back (\"\")"=w253) -> ("States Out"=w258:string)  [unwired: 13 in]
            n90 = call <vilib>:"Add State(s) to Queue__jki_lib_state_machine.vi"("State(s) in Front (\"\")"=w258, "State(s) in (\"\")"=w265) -> ("States Out"=w264:string)  [unwired: 13 in]
          }
          frame "---------- Process ----------" {
            # "Template Separator\n(You can make a copy of, or modify, this frame)"
            n91 = call <vilib>:"Add State(s) to Queue__jki_lib_state_machine.vi"("State(s) in (\"\")"=w270) -> ("States Out"=w269:string)  [unwired: 14 in]
          }
          frame "Process: Sync" {
            n92 = Unbundle By Name(w278) -> ("Self Reference"=w274:refnum<class "SMO.UI.MAUI.BasicTemplate.lvclass">)
            n93 = call <vilib>:"WaitOnProcessSync.vi"("error in (no error)"=w273, "SMO"=w274) -> ("error out"=w272:errorcluster, "Don't run?"=w277:bool)  [unwired: 7 in, 1 out]
            n94 = Select(t="Data: Cleanup\nEvents: Unregister\nExit", s=w277, f="") -> (s? t:f=w271:string)
            n95 = call <vilib>:"Add State(s) to Queue__jki_lib_state_machine.vi"("State(s) in Front (\"\")"=w271, "State(s) in (\"\")"=w281) -> ("States Out"=w280:string)  [unwired: 13 in]
          }
          frame "---------- Events ----------" {
            # "Template Separator\n(You can make a copy of, or modify, this frame)"
            n96 = call <vilib>:"Add State(s) to Queue__jki_lib_state_machine.vi"("State(s) in (\"\")"=w286) -> ("States Out"=w285:string)  [unwired: 14 in]
          }
          frame "Events: Register" {
            # "Expand to add\nmore events"
            n97 = Unbundle By Name(w296) -> ("Self Reference"=w289:refnum<class "SMO.UI.MAUI.BasicTemplate.lvclass">)
            n98 = call <vilib>:"GetProtectedEvents.vi"("SMO"=w289) -> ("error out"=w290:errorcluster, "SMO Protected Events"=w294:T7)  [unwired: 8 in, 1 out]
            n99 = call "SMO.UI.MAUI.GetPublicEvents.vi"("MAUI"=w289) -> ("error out"=w288:errorcluster, "Public Events"=w287:T8)  [unwired: 8 in, 1 out]
            n100 = register-events(w294, w287) -> (reference out=w295:refnum<event-registration>, error out=w291:errorcluster)  [unwired: 2 in]
            n101 = Merge Errors(w293, w291, w290, w288) -> (w292:errorcluster)
            n102 = call <vilib>:"Add State(s) to Queue__jki_lib_state_machine.vi"("State(s) in (\"\")"=w298) -> ("States Out"=w297:string)  [unwired: 14 in]
          }
          frame "Events: Unregister" {
            n103 = Unregister For Events(event registration refnum=w301, error in=w300) -> (error out=w299:errorcluster)
            n104 = call <vilib>:"Clear Errors.vi"("error in (no error)"=w299) -> ()  [unwired: 5 in, 2 out]
            n105 = call <vilib>:"Add State(s) to Queue__jki_lib_state_machine.vi"("State(s) in (\"\")"=w304) -> ("States Out"=w303:string)  [unwired: 14 in]
          }
          frame "---------- Action ----------" {
            n106 = call <vilib>:"Add State(s) to Queue__jki_lib_state_machine.vi"("State(s) in (\"\")"=w309) -> ("States Out"=w308:string)  [unwired: 14 in]
          }
          frame "Action: Notify UI Closed" {
            n107 = Unbundle By Name(w313) -> ("Self Reference"=w312:refnum<class "SMO.UI.MAUI.BasicTemplate.lvclass">)
            n108 = call <vilib>:"Hide.vi"("error in (no error)"=w311, "SMO.UI"=w312) -> ("error out"=w310:errorcluster)  [unwired: 8 in, 1 out]
            n109 = call <vilib>:"Add State(s) to Queue__jki_lib_state_machine.vi"("State(s) in (\"\")"=w316) -> ("States Out"=w315:string)  [unwired: 14 in]
          }
          frame "Action: Template" {
            n110 = Unbundle By Name(w319) -> ("Self Reference"=w317:refnum<class "SMO.UI.MAUI.BasicTemplate.lvclass">)
            n111 = Bundle By Name(cluster=w319, "Self Reference"=w317) -> (w318:T5)
            n112 = call <vilib>:"Add State(s) to Queue__jki_lib_state_machine.vi"("State(s) in (\"\")"=w323) -> ("States Out"=w322:string)  [unwired: 14 in]
          }
          frame "---------- MAUI ----------" {
            # "Left Subpanel is index 0\nRight Subpanel is Index 1"
            n113 = call <vilib>:"Add State(s) to Queue__jki_lib_state_machine.vi"("State(s) in (\"\")"=w328) -> ("States Out"=w327:string)  [unwired: 14 in]
          }
          frame "MAUI: SendPanelData" {
            w336 = T9 {"SubPanel"=refnum, "Ring"=refnum, "Active"=0} ("Panel")
            w338 = 1  # Active
            w340 = 0  # Active
            n114 = Unbundle By Name(w344) -> ("Self Reference"=w335:refnum<class "SMO.UI.MAUI.BasicTemplate.lvclass">)
            n115 = control-ref of="Left Subpanel"() -> (w331:refnum<vi>)
            n116 = control-ref of="Right Subpanel"() -> (w330:refnum<vi>)
            n117 = control-ref of="Left Ring"() -> (w341:refnum<vi>)
            n118 = control-ref of="Right Ring"() -> (w339:refnum<vi>)
            n119 = Bundle(cluster=w336, "SubPanel"=w331, "Ring"=w341, "Active"=w340) -> (w342:T9)
            n120 = Bundle(cluster=w336, "SubPanel"=w330, "Ring"=w339, "Active"=w338) -> (w337:T9)
            n121 = Build Array(w342, w337) -> (w332:T9[])
            n122 = call "WritePanelData.vi"("error in (no error)"=w333, "Panel Data Array"=w332, "MAUI in"=w335) -> ("error out"=w329:errorcluster, "MAUI out"=w334:refnum<class "SMO.UI.MAUI.BasicTemplate.lvclass">)  [unwired: 7 in]
            n123 = Bundle By Name(cluster=w344, "Self Reference"=w334) -> (w343:T5)
            n124 = call <vilib>:"Add State(s) to Queue__jki_lib_state_machine.vi"("State(s) in (\"\")"=w347) -> ("States Out"=w346:string)  [unwired: 14 in]
          }
          frame "MAUI: UpdatePanel" {
            n125 = Decimal String To Number(string=w354) -> (number=w349:i32)  [unwired: 2 in, 1 out]
            n126 = Unbundle By Name(w356) -> ("Self Reference"=w350:refnum<class "SMO.UI.MAUI.BasicTemplate.lvclass">, "MAUI.Active Index"=w348:i32)
            n127 = call "SMO.UI.MAUI.UpdatePanel.vi"("error in (no error)"=w353, "Embedded"=w348, "Panel"=w349, "MAUI"=w350) -> ("error out"=w352:errorcluster, "MAUI out"=w351:refnum<class "SMO.UI.MAUI.BasicTemplate.lvclass">)  [unwired: 6 in]
            n128 = Bundle By Name(cluster=w356, "Self Reference"=w351) -> (w355:T5)
            n129 = call <vilib>:"Add State(s) to Queue__jki_lib_state_machine.vi"("State(s) in (\"\")"=w359) -> ("States Out"=w358:string)  [unwired: 14 in]
          }
        }
      }
    }
    frame Error {
    }
  }
  n130 = call-parent "Process.vi"("error in"=w7, "MAUI"=w1) -> ("error out"=w5:errorcluster, "MAUI out"=→"MauiTemplate out":refnum<class "SMO.UI.MAUI.BasicTemplate.lvclass">)  [unwired: 8 in]
  n131 = Merge Errors(w5, w4) -> (→"error out":errorcluster)
